vi "Set XRT-U Speed.vi"(8 "error in (no error)":errorcluster, 10 "Rate (°/min)":dbl, 11 "Inst.Xeryon-Rotator in":refnum<class "Inst.Xeryon-Rotator.lvclass">) -> (0 "error out":errorcluster, 3 "Inst.Xeryon-Rotator out":refnum<class "Inst.Xeryon-Rotator.lvclass">)   [LabVIEW 2019, in "Inst.Xeryon-Rotator.lvclass"]
uses:
  <userlib>/LevyLab/Xeryon-Rotator/lvsrc/SMOs/Inst.Xeryon-Rotator/Inst.Xeryon-Rotator.lvclass
  <userlib>/LevyLab/Xeryon-Rotator/lvsrc/SMOs/Inst.Xeryon-Rotator/Inst.Xeryon-Rotator.lvclass/Inst.Xeryon-Rotator.ctl
  <userlib>/LevyLab/Xeryon-Rotator/lvsrc/drivers/Class/Controller/Controller.lvclass
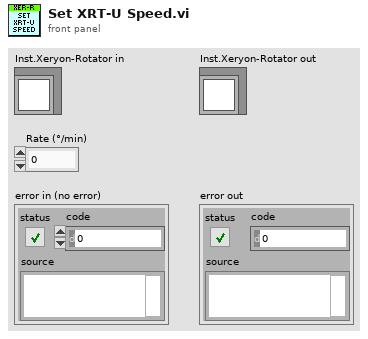
[diagram p1: front panel]
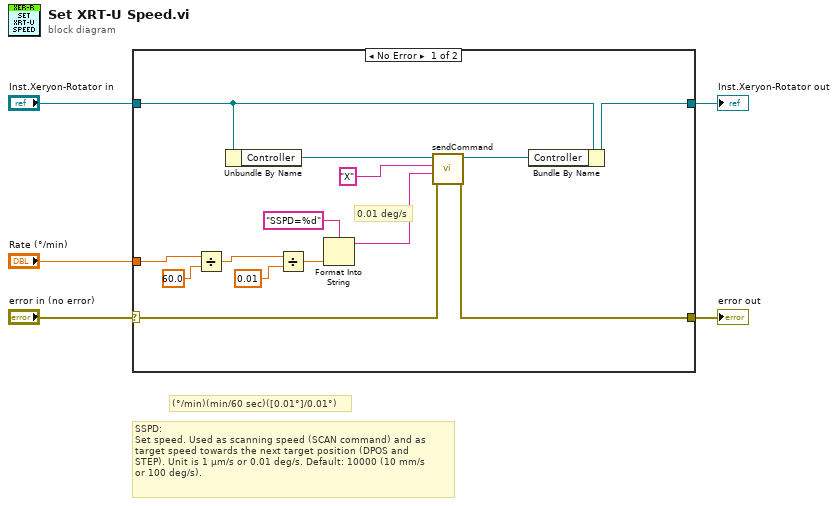
[diagram p0: block diagram]
diagram:
  # "SSPD:\nSet speed. Used as scanning speed (SCAN command) and as\ntarget speed towards the next target position (DPOS and\nSTEP). Unit is 1 µm/s or 0.01 deg/s. Default: 10000 (10 mm/s\nor 100 deg/s)."
  # "(°/min)(min/60 sec)([0.01°]/0.01°)"
  n1 = case shown="No Error" "error in (no error)" {
    selector: "error in (no error)" -> [w6 w21]
    tunnel: [w19 w20] -> w5
    tunnel: "Rate (°/min)" -> [w11 _]
    tunnel: [w9 w21] -> w3
    tunnel: "Inst.Xeryon-Rotator in" -> [w8 w20]
    frame No Error {
      # "0.01 deg/s"
      n2 = Divide(x=w11, y=60.0) -> (x/y=w13:dbl)
      n3 = Unbundle By Name(w8) -> ("Controller"=w17:refnum<class "Controller.lvclass">)
      n4 = Divide(x=w13, y=0.01) -> (x/y=w14:dbl)
      n5 = Format Into String(format string="SSPD=%d", w14) -> (resulting string=w7:string)  [unwired: 2 in, 1 out]
      n6 = call-dynamic "sendCommand.vi"("error in (no error)"=w6, "Command"=w7, "Axis Letter"="X", "Controller in"=w17) -> ("error out"=w9:errorcluster, "Controller out"=w18:refnum<class "Controller.lvclass">)  [unwired: 6 in]
      n7 = Bundle By Name(cluster=w8, "Controller"=w18) -> (w19:refnum<class "Inst.Xeryon-Rotator.lvclass">)
    }
    frame Error {
    }
  }
  "Inst.Xeryon-Rotator out" <- w5
  "error out" <- w3
